vi "destroy events.vi"(11 "MQTT events":T1) -> ()   [LabVIEW 2013, in "MQTT.lvlib"]
uses:
  MQTT.lvlib
  events.ctl
  subMsg.ctl
  statusMsg.ctl
  msgAck.ctl
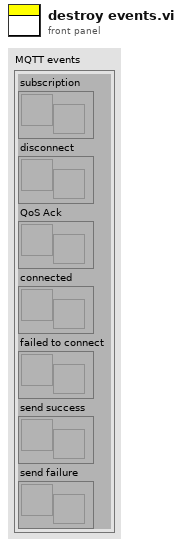
[diagram p1: front panel]
types:
  T1 = typedef "MQTT.lvlib/events.ctl" = cluster{"subscription":refnum<user-event>, "disconnect":refnum<user-event>, "QoS Ack":refnum<user-event>, "connected":refnum<user-event>, "failed to connect":refnum<user-event>, "send success":refnum<user-event>, "send failure":refnum<user-event>}
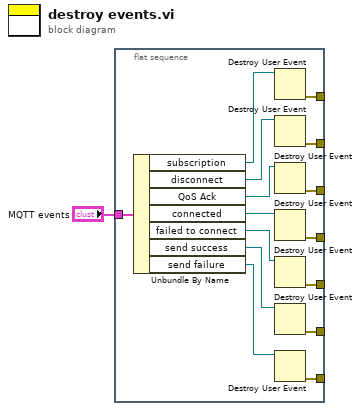
[diagram p0: block diagram]
diagram:
  n1 = flat-sequence {
    tunnel: "MQTT events" -> [w16]
    tunnel: [w14] -> _
    tunnel: [w13] -> _
    tunnel: [w12] -> _
    tunnel: [w11] -> _
    tunnel: [w10] -> _
    tunnel: [w9] -> _
    tunnel: [w8] -> _
    frame #0 {
      n2 = Unbundle By Name(w16) -> ("subscription"=w2:refnum<user-event>, "disconnect"=w3:refnum<user-event>, "QoS Ack"=w4:refnum<user-event>, "connected"=w15:refnum<user-event>, "failed to connect"=w5:refnum<user-event>, "send success"=w6:refnum<user-event>, "send failure"=w7:refnum<user-event>)
      n3 = Destroy User Event(user event=w2) -> (error out=w11:errorcluster)  [unwired: 1 in]
      n4 = Destroy User Event(user event=w3) -> (error out=w12:errorcluster)  [unwired: 1 in]
      n5 = Destroy User Event(user event=w4) -> (error out=w13:errorcluster)  [unwired: 1 in]
      n6 = Destroy User Event(user event=w15) -> (error out=w14:errorcluster)  [unwired: 1 in]
      n7 = Destroy User Event(user event=w5) -> (error out=w10:errorcluster)  [unwired: 1 in]
      n8 = Destroy User Event(user event=w6) -> (error out=w9:errorcluster)  [unwired: 1 in]
      n9 = Destroy User Event(user event=w7) -> (error out=w8:errorcluster)  [unwired: 1 in]
    }
  }
